vi "(SubVI)Scope_Trigger.vi"(6 "Activated Ch":bool[](array[boolean]), 8 "Scope_Trig Level":dbl=1.0 caption="Trigger Level" min=-16.0 max=16.0 format="%#_g g", 9 "Scope_Trig Edge":enum16{"Rising", "Falling"}(ring) caption="Trigger Edge", 10 "Scope_Trig Ch":i32(ring)=-1 caption="Trigger Ch" items=["All Channel"=-1, "Sensor 1 - X"=0, "Sensor 1 - Y"=1, "Sensor 1 - Z"=2, "Sensor 2 - X"=3, "Sensor 2 - Y"=4, "Sensor 2 - Z"=5, "Sensor 3 - X"=6, "Sensor 3 - Y"=7, "Sensor 3 - Z"=8], 11 "data in":dbl[][](array[numeric])) -> (1 "Trigger":bool, 2 "Trigger Point":i32, 3 "data out":dbl[][](array[numeric]))   [LabVIEW 2020]
uses:
  6c56ba6d-c4d1-4d82-9ce7-6f7495d326c9.vi
  6ef858ce-e335-4b38-ab13-2eee3033923d.vi
  <vilib>/Comparison/Equal/Equal Functor/Equal Functor.lvclass
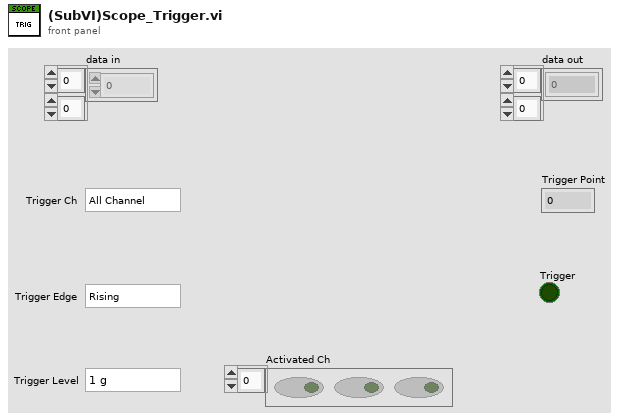
[diagram p1: front panel]
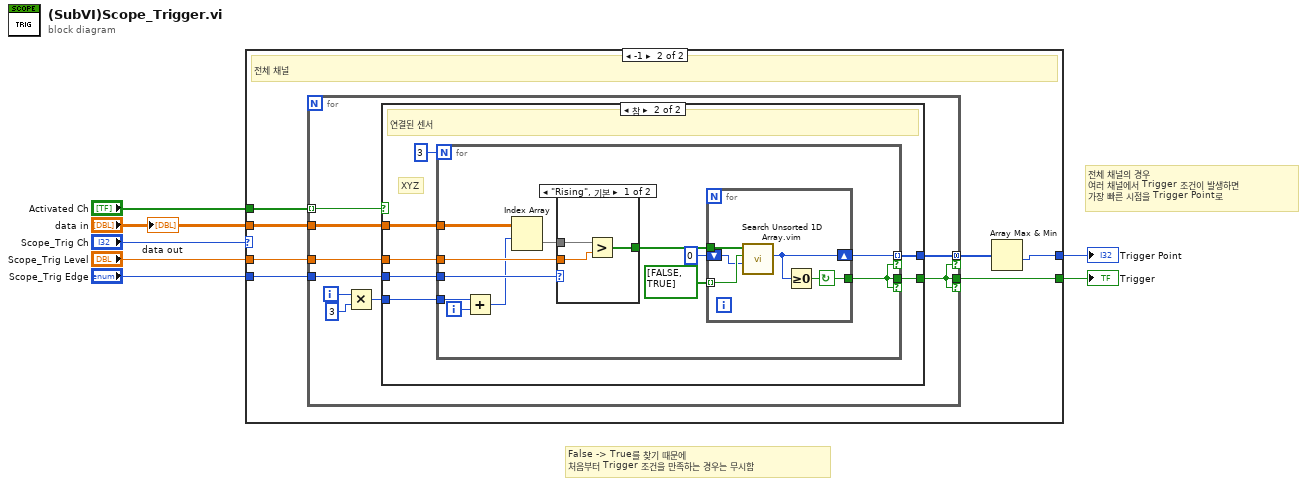
[diagram p0: block diagram]
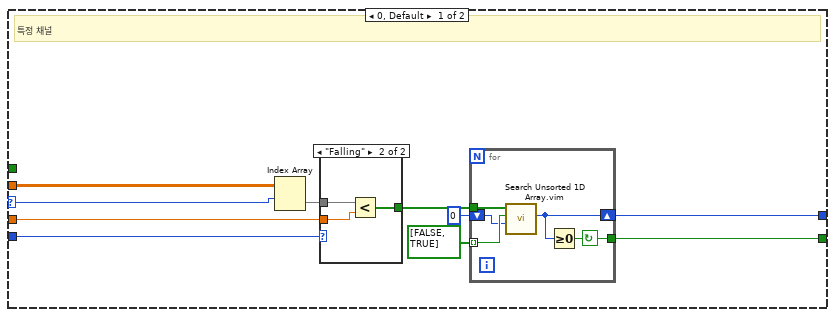
[diagram p2: hidden frame]
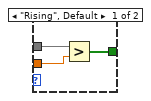
[diagram p3: hidden frame]
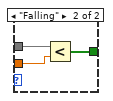
[diagram p5: hidden frame]
diagram:
  # "전체 채널의 경우\n여러 채널에서 Trigger 조건이 발생하면\n가장 빠른 시점을 Trigger Point로"
  # "False -> True를 찾기 때문에 \n처음부터 Trigger 조건을 만족하는 경우는 무시함"
  n1 = case shown="-1" "Scope_Trig Ch" {
    selector: "Scope_Trig Ch" -> [w8 _]
    tunnel: "data in" -> [w17 w35]
    tunnel: "Scope_Trig Edge" -> [w16 w34]
    tunnel: "Scope_Trig Level" -> [w15 w33]
    tunnel: [w10 w29] -> w3
    tunnel: [w9 w31] -> w2
    tunnel: "Activated Ch" -> [_ w30]
    frame 0, Default {
      # "특정 채널"
      n2 = Index Array(array=w17, index (row)=w8) -> (element=w14:dbl[])  [unwired: 1 in]
      n3 = case shown="\"Falling\"" w16 {
        tunnel: w15 -> [w24 w27]
        tunnel: w14 -> [w25 w28]
        tunnel: [w23 w26] -> w13
        frame "Rising", Default {
          n4 = Greater?(x=w25, y=w24) -> (0:w23:bool[])
        }
        frame "Falling" {
          n5 = Less?(x=w28, y=w27) -> (x < y?=w26:bool[])
        }
      }
      n6 = for {
        tunnel: w13 -> [w22]
        tunnel: bool[] [FALSE, TRUE] -> [w21] mode=indexing
        shift-right: [w19] -> w10
        shift-left: 0 ("index of element") -> [w20]
        tunnel: [w18] -> w9
        stop <- w18 continue-if-true
        n7 = call "Search Unsorted 1D Array.vim"("start index (0)"=w20, "element"=w21, "unsorted 1D array"=w22) -> ("index of element"=w19:i32)  [unwired: 8 in]
        n8 = Greater Or Equal To 0?(x=w19) -> (x >= 0?=w18:bool)
      }
    }
    frame -1 {
      # "전체 채널"
      n9 = for {
        tunnel: w35 -> [w44]
        tunnel: w34 -> [w43]
        tunnel: w33 -> [w42]
        tunnel: [w41] -> w32 mode=concatenating if=w36
        tunnel: [w36] -> w31 if=w36
        tunnel: w30 -> [w40] mode=indexing
        i -> [w39]
        n10 = Multiply(x=w39, y=3) -> (x*y=w37:i32)
        n11 = case shown="참" w40 {
          tunnel: w44 -> [_ w51]
          tunnel: w43 -> [_ w50]
          tunnel: w42 -> [_ w49]
          tunnel: [_ w48] -> w41
          tunnel: [_ w46] -> w36
          tunnel: w37 -> [_ w45]
          frame False {
            # "연결되지 않은 센서"
          }
          frame True {
            # "XYZ"
            # "연결된 센서"
            n12 = for {
              N: 3 -> [_]
              tunnel: w51 -> [w57]
              tunnel: w50 -> [w63]
              tunnel: w49 -> [w62]
              tunnel: [w58] -> w48 mode=indexing if=w52
              tunnel: [w52] -> w46 if=w52
              tunnel: w45 -> [w55]
              i -> [w54]
              n13 = Add(x=w55, y=w54) -> (x+y=w53:i32)
              n14 = Index Array(array=w57, index (row)=w53) -> (element=w56:dbl[])  [unwired: 1 in]
              n15 = case shown="\"Rising\", 기본" w63 {
                tunnel: w62 -> [w70 w73]
                tunnel: w56 -> [w71 w74]
                tunnel: [w69 w72] -> w61
                frame "Rising", Default {
                  n16 = Greater?(x=w71, y=w70) -> (0:w69:bool[])
                }
                frame "Falling" {
                  n17 = Less?(x=w74, y=w73) -> (x < y?=w72:bool[])
                }
              }
              n18 = for {
                tunnel: w61 -> [w68]
                tunnel: bool[] [FALSE, TRUE] -> [w67] mode=indexing
                shift-right: [w65] -> w58
                shift-left: 0 ("index of element") -> [w66]
                tunnel: [w64] -> w52
                stop <- w64 continue-if-true
                n19 = call "Search Unsorted 1D Array.vim"("start index (0)"=w66, "element"=w67, "unsorted 1D array"=w68) -> ("index of element"=w65:i32)  [unwired: 8 in]
                n20 = Greater Or Equal To 0?(x=w65) -> (x >= 0?=w64:bool)
              }
            }
          }
        }
      }
      n21 = Array Max & Min(array=w32) -> (min value=w29:i32)  [unwired: 3 out]
    }
  }
  "Trigger Point" <- w3
  "Trigger" <- w2
  "data out" <- "data in"
